vi "Get Data Size.vi"(8 "error in (no error)":errorcluster, 11 "Variant":variant) -> (0 "error out":errorcluster, 2 "ndims":i32, 3 "size":u32[](array[numeric]))   [LabVIEW 2019]
uses:
  <vilib>/Utility/Data Type/Type Definitions/Data Type.ctl
  <vilib>/Utility/Data Type/NI_Data Type.lvlib
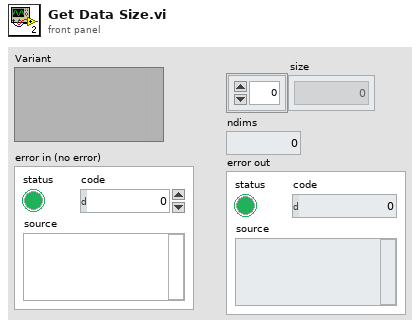
[diagram p1: front panel]
types:
  T1 = typedef "NI_Data Type.lvlib/Data Type.ctl" = enum8{"Invalid Type", "Void", "I8", "I16", "I32", "I64", "U8", "U16", "U32", "U64", "Single Float", "Double Float", "Extended Float", "Single Complex", "Double Complex", "Extended Complex", "Enum U8", "Enum U16", "Enum U32", "Enum U64", "Single Float With Unit", "Double Float With Unit", "Extended Float With Unit", "Single Complex with Unit", "Double Complex with Unit", "Extended Complex with Unit", "Boolean", "String", "Path", "Picture", "Tag", "Array", "Cluster", "Variant", "LV Variant", "Waveform", "Timestamp", "Digital Waveform", "Digital Data", "ExpressData", "Refnum", "External Data", "VI", "Poly VI", "LabVIEW Class Instance", "Fixed Point", "Set Collection", "Map Collection"}
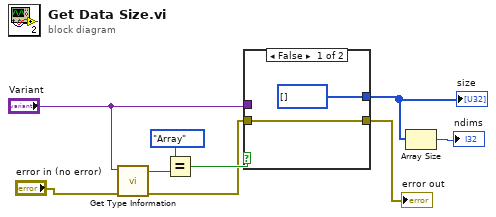
[diagram p0: block diagram]
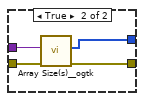
[diagram p2: hidden frame]
diagram:
  n1 = call <vilib>:"Get Type Information.vi"("error in (no error)"="error in (no error)", "variant"="Variant") -> ("error out"=w4:errorcluster, "type"=w8:T1)  [unwired: 5 in, 3 out]
  n2 = Equal?(x=Data_Type."Array", y=w8) -> (x = y?=w7:bool)
  n3 = case shown="False" w7 {
    tunnel: "Variant" -> [_ w14]
    tunnel: w4 -> [w11 w15]
    tunnel: [u32[] [] w12] -> w2
    tunnel: [w11 w13] -> w1
    frame False {
    }
    frame True {
      n4 = call <userlib>:"Array Size(s)__ogtk.vi"("error in (no error)"=w15, "Array"=w14) -> ("error out"=w13:errorcluster, "Size(s)"=w12:u32[])  [unwired: 7 in, 1 out]
    }
  }
  "size" <- w2
  "error out" <- w1
  n5 = Array Size(array=w2) -> (size(s)=→"ndims":i32)
